vi "LuaVIEW Bootstrap Module.vi"(5 "LuaVIEW reference":T1, 7 "function index":i32) -> (15 "error out":errorcluster)   [LabVIEW 2012]
doc: "For documentation of the configuration settings, see the descriptions of the corresponding LabVIEW globals."
uses:
  typedefs/t_LuaVIEW Reference.ctl
  glb_LuaVIEW Configuration Globals.vi
  library/glb_Library Configuration Globals.vi
  LuaVIEW Pull (path).vi
  LuaVIEW Pull (string).vi
  LuaVIEW Pull (flat data).vi
  LuaVIEW Pull (refnum).vi
  LuaVIEW Push (path).vi
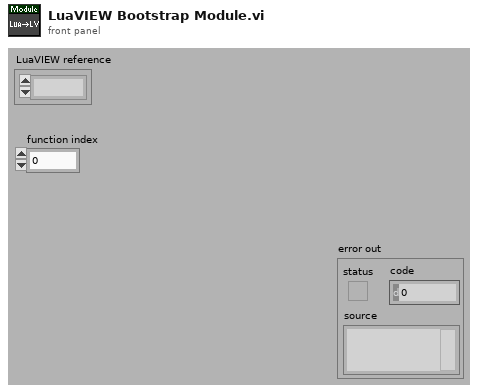
[diagram p1: front panel]
types:
  T1 = typedef "t_LuaVIEW Reference.ctl" = refnum<k1>
  T2 = enum32{"initialize", "configure(tab:configuration)", "configure check", "str:path=bootstrap_path()", "str:path=toolkit_path(str:toolkit,[str:subpath])", "str:kind=app_kind()", "register.public(str:path)", "register.public_dir(str:dirpath)", "do_script(str:name,[str:script])", "cleanup"}
  T3 = cluster{"resource base path":path, "time format":string, "persistence path":path, "bootmode":string, "auto-init registry":bool, "unload functions ASAP":bool, "script search directories":path[], "custom info":string, "export timeout":u32, "incite timeout":u32, "mandatory import script":string, "task error logger":string}
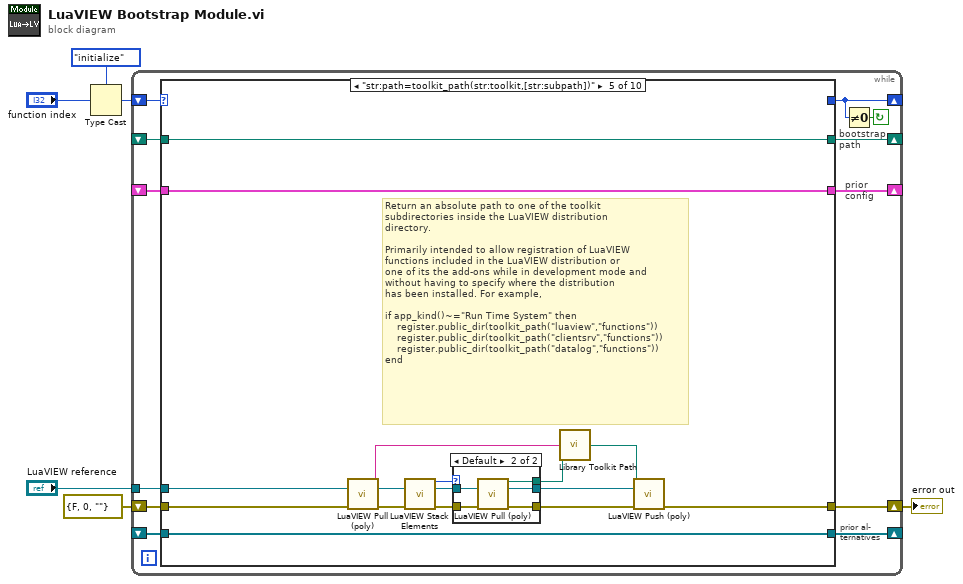
[diagram p0: block diagram]
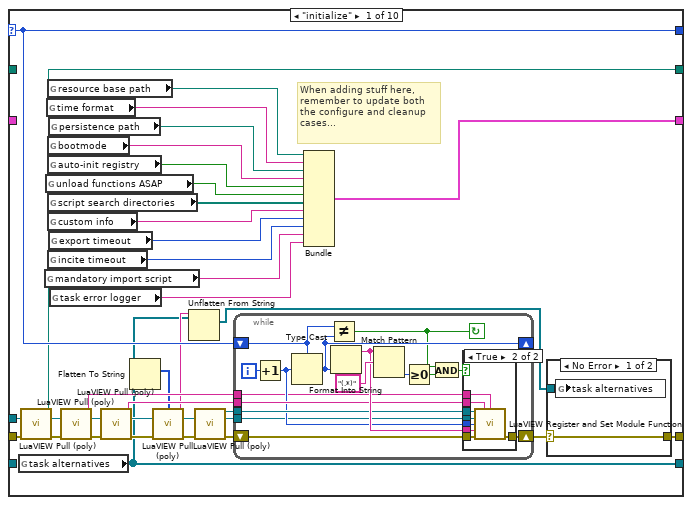
[diagram p2: hidden frame]
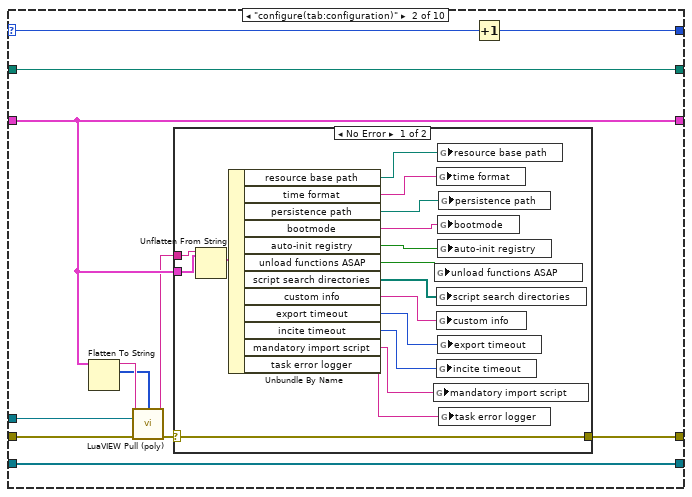
[diagram p5: hidden frame]
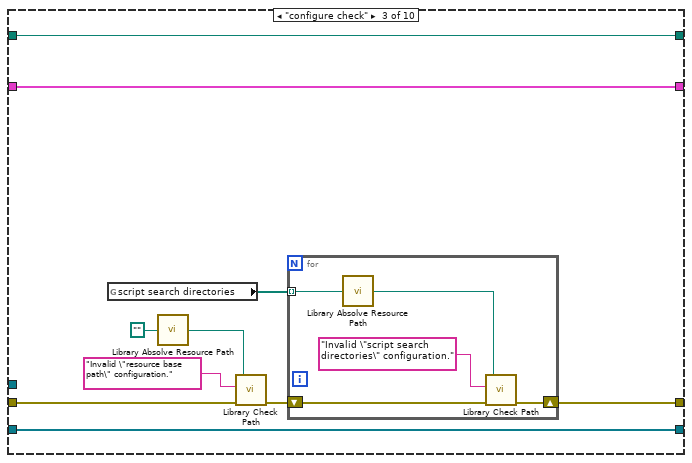
[diagram p7: hidden frame]
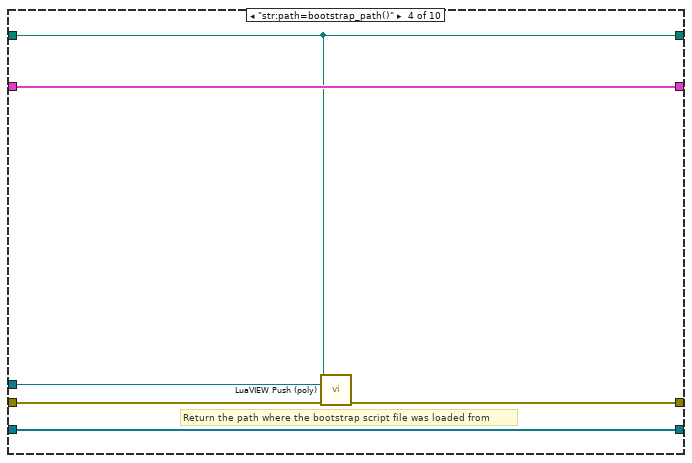
[diagram p8: hidden frame]
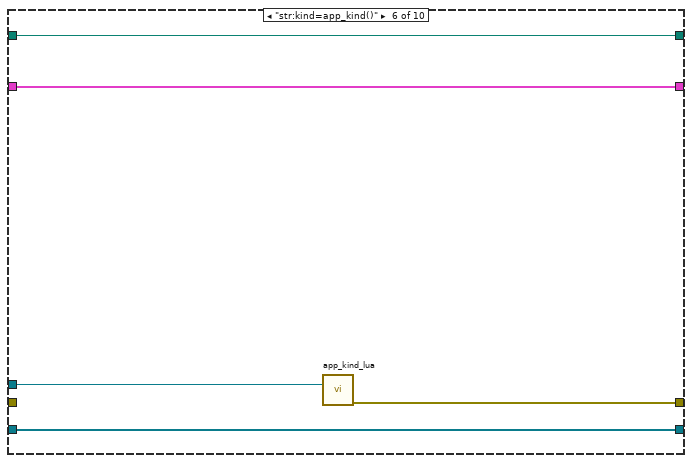
[diagram p10: hidden frame]
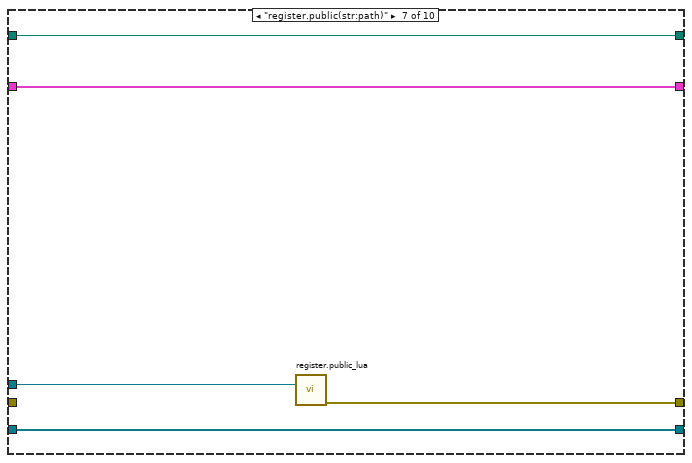
[diagram p11: hidden frame]
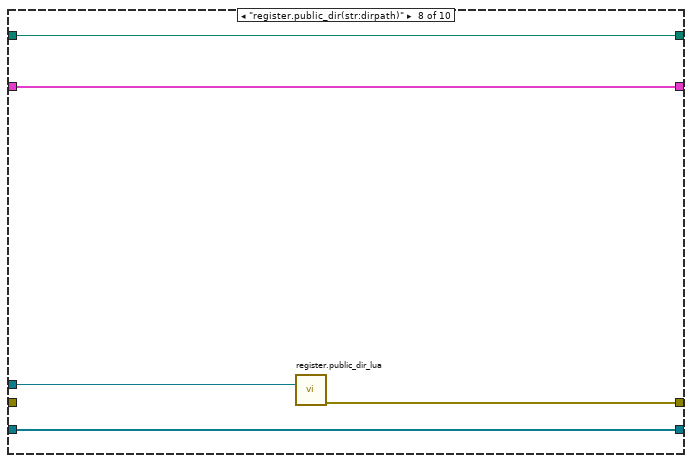
[diagram p12: hidden frame]
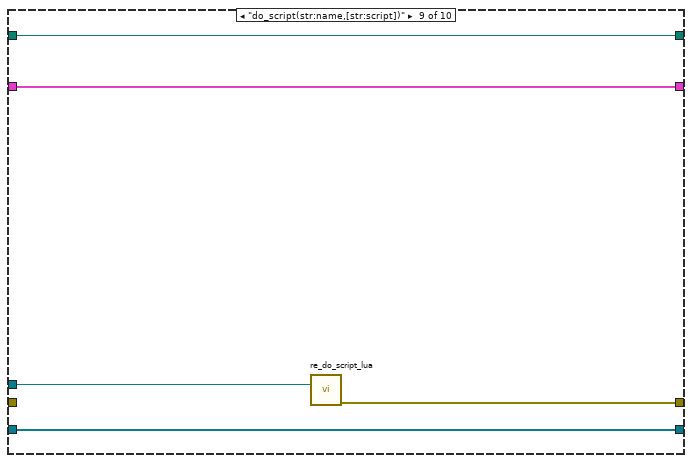
[diagram p13: hidden frame]
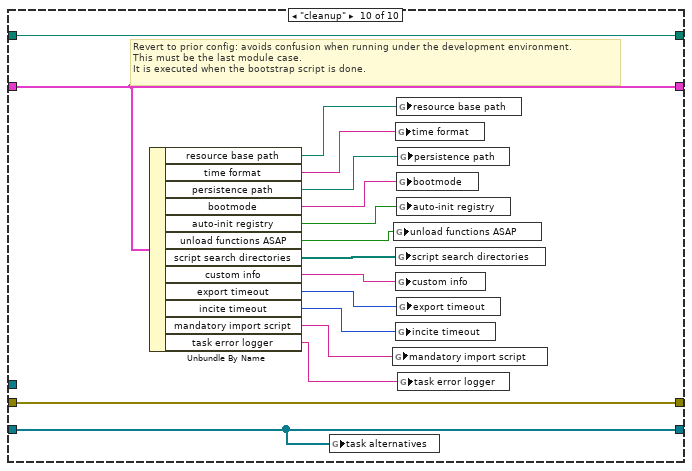
[diagram p14: hidden frame]
diagram:
  n1 = Type Cast(type=T2."initialize", x="function index") -> (*(type *) &x=w4:T2)
  n2 = while {
    shift-right: [w12] -> _
    shift-left: w4 -> [w18]
    shift-right: [w17] -> w6
    shift-left: errorcluster {"status"=FALSE, "code"=0, "source"=""} ("error out") -> [w16]
    shift-right: [w13] -> _
    shift-left: _ -> [w15]
    tunnel: "LuaVIEW reference" -> [w14]
    shift-right: [w10] -> _
    shift-left: _ -> [w9]
    shift-right: [w8] -> _
    shift-left: _ -> [w7]
    stop <- w11 continue-if-true
    # "prior al-\nternatives"
    # "bootstrap\npath"
    # "prior\nconfig"
    n3 = case shown="\"str:path=toolkit_path(str:toolkit,[str:subpath])\"" w18 {
      selector: w18 -> [w54 w87 _ _ _ _ _ _ _ _]
      tunnel: [w54 w86 _ _ _ _ _ _ _ _] -> w12
      tunnel: w14 -> [w35 w93 _ w131 w144 w158 w164 w169 w173 _]
      tunnel: [w22 w84 w113 w128 w140 w159 w163 w168 w174 w191] -> w17
      tunnel: w16 -> [w34 w94 w117 w130 w145 _ _ _ _ w191]
      tunnel: w15 -> [_ w90 w121 w132 w148 w160 w165 w170 w175 w190]
      tunnel: [w53 w90 w121 w132 w148 w160 w165 w170 w175 w190] -> w13
      tunnel: [w33 w88 w120 w129 w147 w157 w162 w167 w172 w181] -> w10
      tunnel: w9 -> [_ w88 w120 w129 w147 w157 w162 w167 w172 w181]
      tunnel: [w24 w83 w112 w127 w146 w156 w161 w166 w171 w178] -> w8
      tunnel: w7 -> [_ w83 w112 w127 w146 w156 w161 w166 w171 w178]
      frame "initialize" {
        # "When adding stuff here,\nremember to update both\nthe configure and cleanup\ncases..."
        n4 = global read "glb_LuaVIEW Configuration Globals.vi" "task alternatives"() -> (w24:refnum<vi>[])
        n5 = call-poly "LuaVIEW Pull (poly).vi"("LuaVIEW reference in"=w35, "error in (no error)"=w34) -> ("path"=w33:path, "LuaVIEW reference out"=w37:T1, "error out"=w36:errorcluster)  [unwired: 11 in]
        n6 = global read "glb_LuaVIEW Configuration Globals.vi" "mandatory import script"() -> (w31:string)
        n7 = global read "glb_LuaVIEW Configuration Globals.vi" "unload functions ASAP"() -> (w44:bool)
        n8 = global read "glb_Library Configuration Globals.vi" "time format"() -> (w39:string)
        n9 = global read "glb_Library Configuration Globals.vi" "resource base path"() -> (w40:path)
        n10 = global read "glb_LuaVIEW Configuration Globals.vi" "bootmode"() -> (w20:string)
        n11 = global read "glb_LuaVIEW Configuration Globals.vi" "auto-init registry"() -> (w45:bool)
        n12 = global read "glb_LuaVIEW Configuration Globals.vi" "script search directories"() -> (w43:path[])
        n13 = global read "glb_LuaVIEW Configuration Globals.vi" "custom info"() -> (w42:string)
        n14 = global read "glb_LuaVIEW Configuration Globals.vi" "incite timeout"() -> (w32:u32)
        n15 = global read "glb_Library Configuration Globals.vi" "persistence path"() -> (w38:path)
        n16 = global read "glb_LuaVIEW Configuration Globals.vi" "export timeout"() -> (w41:u32)
        n17 = global read "glb_LuaVIEW Configuration Globals.vi" "task error logger"() -> (w19:string)
        n18 = call-poly "LuaVIEW Pull (poly).vi"("LuaVIEW reference in"=w37, "error in (no error)"=w36) -> ("string"=w46:string, "LuaVIEW reference out"=w48:T1, "error out"=w47:errorcluster)  [unwired: 11 in]
        n19 = call-poly "LuaVIEW Pull (poly).vi"("LuaVIEW reference in"=w48, "error in (no error)"=w47) -> ("string"=w51:string, "LuaVIEW reference out"=w29:T1, "error out"=w30:errorcluster)  [unwired: 11 in]
        n20 = Flatten To String(anything=w24) -> (type string=w26:i16[])  [unwired: 3 in, 2 out]
        n21 = call-poly "LuaVIEW Pull (poly).vi"("type descriptor"=w26, "LuaVIEW reference in"=w29, "error in (no error)"=w30) -> ("flat data"=w25:string, "LuaVIEW reference out"=w28:T1, "error out"=w27:errorcluster)  [unwired: 10 in]
        n22 = Unflatten From String(type=w24, binary string=w25) -> (value=w21:refnum<vi>[])  [unwired: 3 in, 2 out]
        n23 = call-poly "LuaVIEW Pull (poly).vi"("LuaVIEW reference in"=w28, "error in (no error)"=w27) -> ("refnum"=w50:refnum<vi>, "LuaVIEW reference out"=w49:T1, "error out"=w52:errorcluster)  [unwired: 11 in]
        n24 = while {
          shift-right: [w70] -> w23
          shift-left: w52 -> [w71]
          shift-right: [w66] -> _
          shift-left: w54 -> [w67]
          tunnel: w50 -> [w65]
          tunnel: w51 -> [w64]
          tunnel: w49 -> [w62]
          tunnel: w46 -> [w61]
          i -> [w69]
          stop <- w58 continue-if-true
          n25 = Increment(x=w69) -> (x+1=w63:i32)
          n26 = Type Cast(type=w67, x=w63) -> (*(type *) &x=w66:T2)
          n27 = Not Equal?(x=w67, y=w66) -> (x != y?=w58:bool)
          n28 = Format Into String(w66) -> (resulting string=w68:string)  [unwired: 3 in, 1 out]
          n29 = Match Pattern(string=w68, regular expression="(.*)") -> (offset past match=w72:i32)  [unwired: 1 in, 3 out]
          n30 = Greater Or Equal To 0?(x=w72) -> (x >= 0?=w60:bool)
          n31 = And(x=w58, y=w60) -> (x .and. y?=w59:bool)
          n32 = case shown="True" w59 {
            tunnel: w62 -> [_ w80]
            tunnel: w63 -> [_ w81]
            tunnel: w68 -> [_ w78]
            tunnel: [w74 w82] -> w70
            tunnel: w71 -> [w74 w79]
            tunnel: w65 -> [_ w77]
            tunnel: w64 -> [_ w76]
            tunnel: w61 -> [_ w75]
            frame False {
            }
            frame True {
              n33 = call "LuaVIEW Register and Set Module Function.vi"("module refnum"=w77, "export table (set as global)"=w76, "table (set as global)"=w75, "LuaVIEW reference in"=w80, "index"=w81, "synopsis"=w78, "error in (no error)"=w79) -> ("error out"=w82:errorcluster)  [unwired: 7 in, 1 out]
            }
          }
        }
        n34 = Bundle("resource base path"=w40, "time format"=w39, "persistence path"=w38, "bootmode"=w20, "auto-init registry"=w45, "unload functions ASAP"=w44, "script search directories"=w43, "custom info"=w42, "export timeout"=w41, "incite timeout"=w32, "mandatory import script"=w31, "task error logger"=w19) -> (w53:T3)  [unwired: 1 in]
        n35 = case shown="No Error" w23 {
          selector: w23 -> [w56 w57]
          tunnel: [w56 w57] -> w22
          tunnel: w21 -> [w55 _]
          frame No Error {
            n36 = global write "glb_LuaVIEW Configuration Globals.vi" "task alternatives"(w55) -> ()
          }
          frame Error {
          }
        }
      }
      frame "configure(tab:configuration)" {
        n37 = Flatten To String(anything=w90) -> (data string=w92:string, type string=w91:i16[])  [unwired: 3 in, 1 out]
        n38 = call-poly "LuaVIEW Pull (poly).vi"("default flat data"=w92, "type descriptor"=w91, "LuaVIEW reference in"=w93, "error in (no error)"=w94) -> ("flat data"=w89:string, "error out"=w85:errorcluster)  [unwired: 9 in, 1 out]
        n39 = case shown="No Error" w85 {
          selector: w85 -> [w97 w111]
          tunnel: w90 -> [w110 _]
          tunnel: w89 -> [w109 _]
          tunnel: [w97 w111] -> w84
          frame No Error {
            n40 = Unflatten From String(type=w110, binary string=w109) -> (value=w100:T3)  [unwired: 3 in, 2 out]
            n41 = Unbundle By Name(w100) -> ("resource base path"=w108:path, "time format"=w107:string, "persistence path"=w106:path, "bootmode"=w96:string, "auto-init registry"=w105:bool, "unload functions ASAP"=w104:bool, "script search directories"=w103:path[], "custom info"=w102:string, "export timeout"=w101:u32, "incite timeout"=w99:u32, "mandatory import script"=w98:string, "task error logger"=w95:string)
            n42 = global write "glb_LuaVIEW Configuration Globals.vi" "mandatory import script"(w98) -> ()
            n43 = global write "glb_LuaVIEW Configuration Globals.vi" "unload functions ASAP"(w104) -> ()
            n44 = global write "glb_Library Configuration Globals.vi" "time format"(w107) -> ()
            n45 = global write "glb_LuaVIEW Configuration Globals.vi" "script search directories"(w103) -> ()
            n46 = global write "glb_LuaVIEW Configuration Globals.vi" "custom info"(w102) -> ()
            n47 = global write "glb_LuaVIEW Configuration Globals.vi" "incite timeout"(w99) -> ()
            n48 = global write "glb_Library Configuration Globals.vi" "resource base path"(w108) -> ()
            n49 = global write "glb_LuaVIEW Configuration Globals.vi" "bootmode"(w96) -> ()
            n50 = global write "glb_LuaVIEW Configuration Globals.vi" "auto-init registry"(w105) -> ()
            n51 = global write "glb_LuaVIEW Configuration Globals.vi" "export timeout"(w101) -> ()
            n52 = global write "glb_Library Configuration Globals.vi" "persistence path"(w106) -> ()
            n53 = global write "glb_LuaVIEW Configuration Globals.vi" "task error logger"(w95) -> ()
          }
          frame Error {
          }
        }
        n54 = Increment(x=w87) -> (x+1=w86:T2)
      }
      frame "configure check" {
        n55 = global read "glb_LuaVIEW Configuration Globals.vi" "script search directories"() -> (w114:path[])
        n56 = call "Library Absolve Resource Path.vi"("path in"=path "") -> ("absolved path"=w118:path)  [unwired: 14 in]
        n57 = call "Library Check Path.vi"("error in (no error)"=w117, "further explanation (none)"="Invalid \"resource base path\" configuration.", "path"=w118) -> ("error out"=w115:errorcluster)  [unwired: 3 in, 1 out]
        n58 = for {
          shift-right: [w124] -> w113
          shift-left: w115 -> [w125]
          tunnel: w114 -> [w126] mode=indexing
          n59 = call "Library Absolve Resource Path.vi"("path in"=w126) -> ("absolved path"=w123:path)  [unwired: 14 in]
          n60 = call "Library Check Path.vi"("error in (no error)"=w125, "further explanation (none)"="Invalid \"script search directories\" configuration.", "path"=w123) -> ("error out"=w124:errorcluster)  [unwired: 3 in, 1 out]
        }
      }
      frame "str:path=bootstrap_path()" {
        # "Return the path where the bootstrap script file was loaded from"
        n61 = call-poly "LuaVIEW Push (poly).vi"("path"=w129, "LuaVIEW reference in"=w131, "error in (no error)"=w130) -> ("error out"=w128:errorcluster)  [unwired: 11 in, 1 out]
      }
      frame "str:path=toolkit_path(str:toolkit,[str:subpath])" {
        # "Return an absolute path to one of the toolkit\nsubdirectories inside the LuaVIEW distribution\ndirectory.\n\nPrimarily intended to allow registration of LuaVIEW\nfunctions included in the LuaVIEW distribution or\none of its the add-ons while in development mode and\nwithout having to specify where the distribution\nhas been installed. For example,\n\nif app_kind()~=\"Run Time System\" then\n    register.public_dir(toolkit_path(\"luaview\",\"functions\"))\n    register.public_dir(toolkit_path(\"clientsrv\",\"functions\"))\n    register.public_dir(toolkit_path(\"datalog\",\"functions\"))\nend"
        n62 = call-poly "LuaVIEW Pull (poly).vi"("LuaVIEW reference in"=w144, "error in (no error)"=w145) -> ("string"=w143:string, "LuaVIEW reference out"=w134:T1, "error out"=w137:errorcluster)  [unwired: 11 in]
        n63 = call "LuaVIEW Stack Elements.vi"("LuaVIEW reference in"=w134, "error in (no error)"=w137) -> ("elements"=w133:i32, "LuaVIEW reference out"=w135:T1, "error out"=w136:errorcluster)  [unwired: 11 in]
        n64 = case shown="Default" w133 {
          tunnel: [_ w155] -> w142
          tunnel: [w149 w154] -> w141
          tunnel: [w150 w153] -> w139
          tunnel: w136 -> [w149 w152]
          tunnel: w135 -> [w150 w151]
          frame 0 {
          }
          frame Default {
            n65 = call-poly "LuaVIEW Pull (poly).vi"("LuaVIEW reference in"=w151, "error in (no error)"=w152) -> ("path"=w155:path, "LuaVIEW reference out"=w153:T1, "error out"=w154:errorcluster)  [unwired: 11 in]
          }
        }
        n66 = call "Library Toolkit Path.vi"("toolkit directory (none)"=w143, "sub path of toolkit (none)"=w142) -> ("absolute toolkit path"=w138:path)  [unwired: 13 in]
        n67 = call-poly "LuaVIEW Push (poly).vi"("path"=w138, "LuaVIEW reference in"=w139, "error in (no error)"=w141) -> ("error out"=w140:errorcluster)  [unwired: 11 in, 1 out]
      }
      frame "str:kind=app_kind()" {
        n68 = call "app_kind_lua.vi"("LuaVIEW reference"=w158) -> ("error out"=w159:errorcluster)  [unwired: 14 in]
      }
      frame "register.public(str:path)" {
        n69 = call "register.public_lua.vi"("LuaVIEW reference"=w164) -> ("error out"=w163:errorcluster)  [unwired: 14 in]
      }
      frame "register.public_dir(str:dirpath)" {
        n70 = call "register.public_dir_lua.vi"("LuaVIEW reference"=w169) -> ("error out"=w168:errorcluster)  [unwired: 14 in]
      }
      frame "do_script(str:name,[str:script])" {
        n71 = call "re_do_script_lua.vi"("LuaVIEW reference"=w173) -> ("error out"=w174:errorcluster)  [unwired: 14 in]
      }
      frame "cleanup" {
        # "Revert to prior config: avoids confusion when running under the development environment.\nThis must be the last module case.\nIt is executed when the bootstrap script is done."
        n72 = Unbundle By Name(w190) -> ("resource base path"=w189:path, "time format"=w188:string, "persistence path"=w187:path, "bootmode"=w176:string, "auto-init registry"=w186:bool, "unload functions ASAP"=w185:bool, "script search directories"=w184:path[], "custom info"=w183:string, "export timeout"=w182:u32, "incite timeout"=w180:u32, "mandatory import script"=w179:string, "task error logger"=w177:string)
        n73 = global write "glb_LuaVIEW Configuration Globals.vi" "task alternatives"(w178) -> ()
        n74 = global write "glb_LuaVIEW Configuration Globals.vi" "mandatory import script"(w179) -> ()
        n75 = global write "glb_LuaVIEW Configuration Globals.vi" "unload functions ASAP"(w185) -> ()
        n76 = global write "glb_Library Configuration Globals.vi" "time format"(w188) -> ()
        n77 = global write "glb_LuaVIEW Configuration Globals.vi" "script search directories"(w184) -> ()
        n78 = global write "glb_LuaVIEW Configuration Globals.vi" "custom info"(w183) -> ()
        n79 = global write "glb_LuaVIEW Configuration Globals.vi" "incite timeout"(w180) -> ()
        n80 = global write "glb_Library Configuration Globals.vi" "resource base path"(w189) -> ()
        n81 = global write "glb_LuaVIEW Configuration Globals.vi" "bootmode"(w176) -> ()
        n82 = global write "glb_LuaVIEW Configuration Globals.vi" "auto-init registry"(w186) -> ()
        n83 = global write "glb_LuaVIEW Configuration Globals.vi" "export timeout"(w182) -> ()
        n84 = global write "glb_Library Configuration Globals.vi" "persistence path"(w187) -> ()
        n85 = global write "glb_LuaVIEW Configuration Globals.vi" "task error logger"(w177) -> ()
      }
    }
    n86 = Not Equal To 0?(x=w12) -> (x != 0?=w11:bool)
  }
  "error out" <- w6
